vi "Reset.vi"(0 "eye scan point iterator":refnum<class "niHighSpeedSerial Rectangular Eye Scan Point Iterator v1 Host.lvclass">, 11 "error in":errorcluster) -> (4 "eye scan point iterator out":refnum<class "niHighSpeedSerial Rectangular Eye Scan Point Iterator v1 Host.lvclass">, 15 "error out":errorcluster)   [LabVIEW 2014, in "niHighSpeedSerial Rectangular Eye Scan Point Iterator v1 Host.lvclass"]
doc: "Puts the Eye Scan Point Iterator back into its initial state, discarding any previous information.\n\n<B>Input Parameters</B>\n\n<B>eye scan point iterator</B> is the incoming wire for the Eye Scan Point Iterator class object\n\n<B>error in</B> describes error conditions that occur before this node runs. This input provides standard 'error in' functionality.\n\n<B>Output Parameters</B>\n\n<B>eye scan point iterator out</B> is the outgoing wire for the Eye Scan Point Iterator class object\n\n<B>error out</B> contains error information. This output provides standard 'error out' functionality."
uses:
  <instrlib>/niHighSpeedSerial/Eye Scan/v1/Host/Impl/Rect Iter/niHighSpeedSerial Rectangular Eye Scan Point Iterator v1 Host.lvclass
  <instrlib>/niHighSpeedSerial/Eye Scan/v1/Host/Impl/Rect Iter/niHighSpeedSerial Rectangular Eye Scan Point Iterator v1 Host.lvclass/niHighSpeedSerial Rectangular Eye Scan Point Iterator v1 Host.ctl
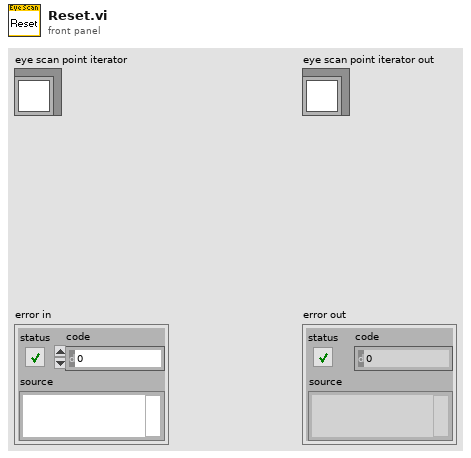
[diagram p1: front panel]
types:
  T1 = typedef "niHighSpeedSerial Eye Scan Common v1 Host.lvlib/Point.ctl" = cluster{"point offsets":T2, "sample count":u64, "error count":u64, "bit error rate":dbl}
  T2 = typedef "niHighSpeedSerial Eye Scan Common v1 Host.lvlib/Point Offsets.ctl" = cluster{"horizontal offset":i16, "vertical offset":i8}
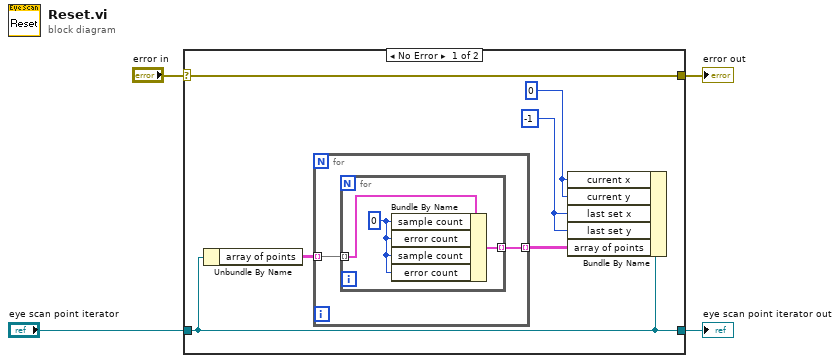
[diagram p0: block diagram]
diagram:
  n1 = case shown="No Error" "error in" {
    selector: "error in" -> [w10 w17]
    tunnel: [w10 w17] -> w3
    tunnel: "eye scan point iterator" -> [w7 w16]
    tunnel: [w7 w16] -> w1
    frame No Error {
      w5 = -1 ("y")
      w6 = 0 ("Current Point Offset In Array")
      n2 = Unbundle By Name(w7) -> ("array of points"=w9:T1[][])
      n3 = for {
        tunnel: w9 -> [w12] mode=indexing
        tunnel: [w11] -> w8 mode=indexing
        n4 = for {
          tunnel: w12 -> [w15] mode=indexing
          tunnel: [w14] -> w11 mode=indexing
          w13 = u64 0 ("sample count")
          n5 = Bundle By Name(cluster=w15, "sample count"=w13, "error count"=w13, "sample count"=w13, "error count"=w13) -> (w14:T1)
        }
      }
      n6 = Bundle By Name(cluster=w7, "current x"=w6, "current y"=w6, "last set x"=w5, "last set y"=w5, "array of points"=w8) -> ()  [unwired: 1 out]
    }
    frame Error {
    }
  }
  "eye scan point iterator out" <- w1
  "error out" <- w3
